vi "Read Succeed State .vi"(8 "error in (no error)":errorcluster, 11 "abs_Test Boolean in":refnum<class "abs_Test Boolean.lvclass">) -> (0 "error out":errorcluster, 2 "Succeed State":T1, 3 "abs_Test Boolean out":refnum<class "abs_Test Boolean.lvclass">)   [LabVIEW 2021, in "BT.lvlib" / "abs_Test Boolean.lvclass"]
uses:
  abs_Test Boolean.lvclass
  Support/Succeed State.ctl
  abs_Test Boolean.lvclass/abs_Test Boolean.ctl
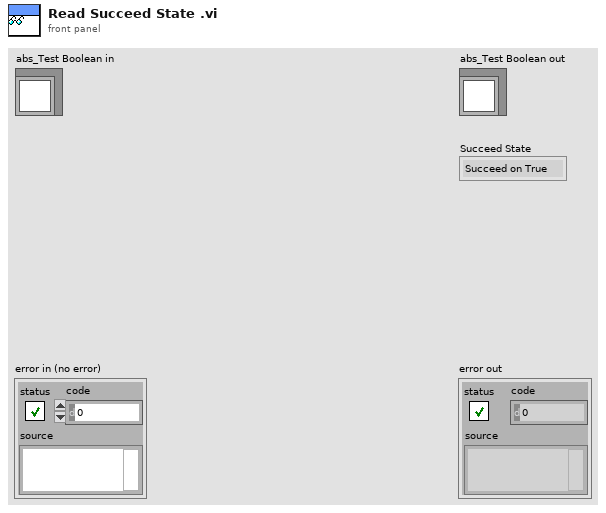
[diagram p1: front panel]
types:
  T1 = typedef "BT.lvlib/abs_Test Boolean.lvclass/Succeed State.ctl" = enum16{"Succeed on True", "Succeed on Fail"}
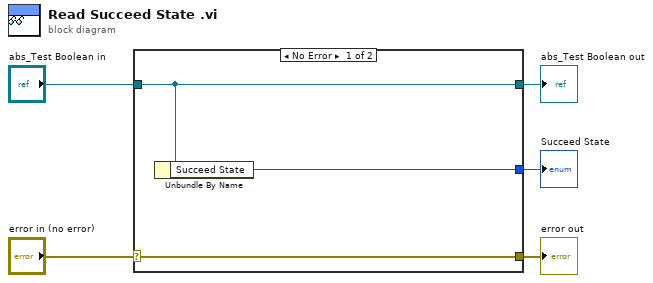
[diagram p0: block diagram]
diagram:
  n1 = case shown="No Error" "error in (no error)" {
    selector: "error in (no error)" -> [w8 w9]
    tunnel: [w8 w9] -> w4
    tunnel: [w7 w10] -> w2
    tunnel: "abs_Test Boolean in" -> [w7 w10]
    tunnel: [w6 _] -> w1
    frame No Error {
      n2 = Unbundle By Name(w7) -> ("Succeed State"=w6:T1)
    }
    frame Error {
    }
  }
  "error out" <- w4
  "abs_Test Boolean out" <- w2
  "Succeed State" <- w1
